vi "2feladat.vi"() -> ()   [LabVIEW 2016]
panel:
  out "Numeric 2":dbl
  in  "Numeric":dbl
  out "Boolean 2":bool
  in  "Boolean":bool
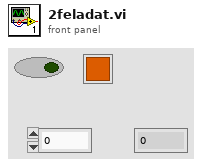
[diagram p1: front panel]
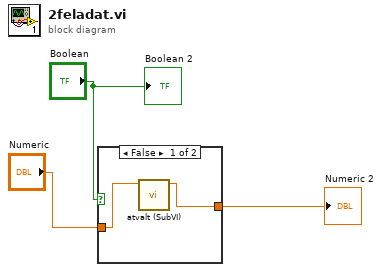
[diagram p0: block diagram]
diagram:
  n1 = case shown="False" "Boolean" {
    tunnel: "Numeric" -> [w5 w6]
    tunnel: [w4 w6] -> w1
    frame False {
      n2 = call "atvalt (SubVI).vi"("Numeric in"=w5) -> ("Numeric out"=w4:dbl)  [unwired: 10 in]
    }
    frame True {
    }
  }
  "Numeric 2" <- w1
  "Boolean 2" <- "Boolean"
